vi "test_MultipleStartStopSMO.vi"(8 "error in (no error)":errorcluster, 11 "TestCase in":refnum<class "SMO_TestCase.lvclass">) -> (0 "error out":errorcluster, 3 "TestCase out":refnum<class "SMO_TestCase.lvclass">)   [LabVIEW 2013, in "SMO_TestCase.lvclass"]
uses:
  SMO_TestCase.lvclass
  SMO_TestCase.lvclass/SMO_TestCase.ctl
  <vilib>/addons/_JKI Toolkits/VI Tester/TestCase.llb/TestCase.lvclass
  Projects/JKI SMO Git/JKI-State-Machine-Objects/src/SMO/SMO.lvclass
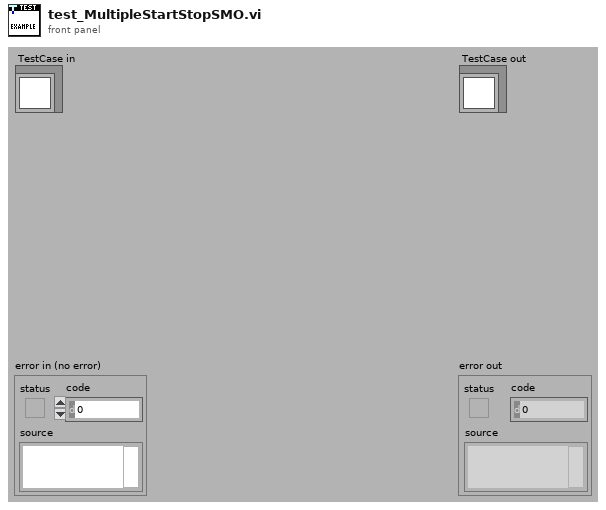
[diagram p1: front panel]
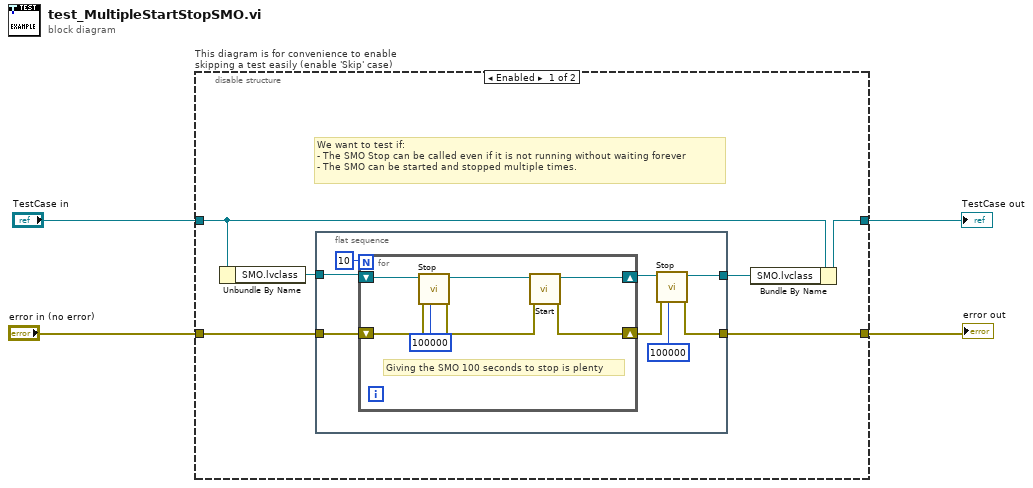
[diagram p0: block diagram]
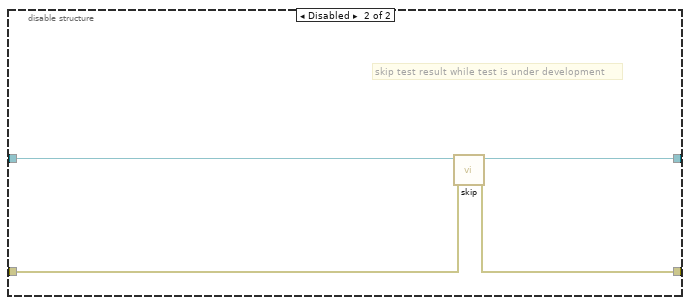
[diagram p2: hidden frame]
diagram:
  n1 = disable-structure "This diagram is for convenience to enable skipping a test easily (enable 'Skip' case)" shown="Enabled" {
    disable-tunnel: "TestCase in" -> [w8 w29]
    disable-tunnel: [w7 w27] -> w1
    disable-tunnel: [w5 w28] -> w3
    disable-tunnel: "error in (no error)" -> [w9 w26]
    frame Enabled {
      # "We want to test if:\n- The SMO Stop can be called even if it is not running without waiting forever\n- The SMO can be started and stopped multiple times."
      n2 = Unbundle By Name(w8) -> ("SMO.lvclass"=w10:refnum<class "SMO.lvclass">)
      n3 = flat-sequence {
        tunnel: w10 -> [w18]
        tunnel: w9 -> [w17]
        tunnel: [w14] -> w6
        tunnel: [w12] -> w5
        frame #0 {
          n4 = for {
            N: 10 -> [_]
            shift-right: [w21] -> w15
            shift-left: w18 -> [w24]
            shift-right: [w19] -> w13
            shift-left: w17 -> [w23]
            # "Giving the SMO 100 seconds to stop is plenty"
            n5 = call "Stop.vi"("timeout in ms (-1)"=100000, "error in (no error)"=w23, "SMO"=w24) -> ("error out"=w20:errorcluster, "SMO out"=w22:refnum<class "SMO.lvclass">)  [unwired: 7 in]
            n6 = call "Start.vi"("error in (no error)"=w20, "SMO"=w22) -> ("error out"=w19:errorcluster, "SMO out"=w21:refnum<class "SMO.lvclass">)  [unwired: 8 in]
          }
          n7 = call "Stop.vi"("timeout in ms (-1)"=100000, "error in (no error)"=w13, "SMO"=w15) -> ("error out"=w12:errorcluster, "SMO out"=w14:refnum<class "SMO.lvclass">)  [unwired: 7 in]
        }
      }
      n8 = Bundle By Name(cluster=w8, "SMO.lvclass"=w6) -> (w7:refnum<class "SMO_TestCase.lvclass">)
    }
    frame Disabled {
      # "skip test result while test is under development"
      n9 = call <vilib>:"skip.vi"("error in (no error)"=w26, "TestCase in"=w29) -> ("error out"=w28:errorcluster, "TestCase out"=w27:refnum<class "SMO_TestCase.lvclass">)  [unwired: 8 in]
    }
  }
  "error out" <- w3
  "TestCase out" <- w1
